vi "getlastmondata.vi"(0 "duplicate VISA resource name":refnum<visa-resource-name>, 1 "error out 2":errorcluster) -> (2 "duplicate VISA resource name 2":refnum<visa-resource-name>, 3 "output cluster":T1, 4 "N":u16, 5 "error out":errorcluster)   [LabVIEW 2010]
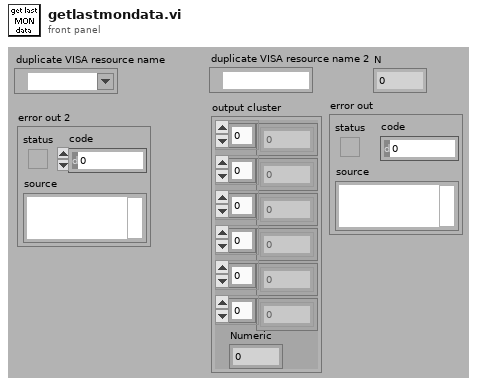
[diagram p1: front panel]
types:
  T1 = cluster{u16[], u16[], u16[], u16[], u16[], u16[], "Numeric":dbl}
  T2 = cluster{u16[], u16[], u16[], u16[], u16[], u16[], u16}
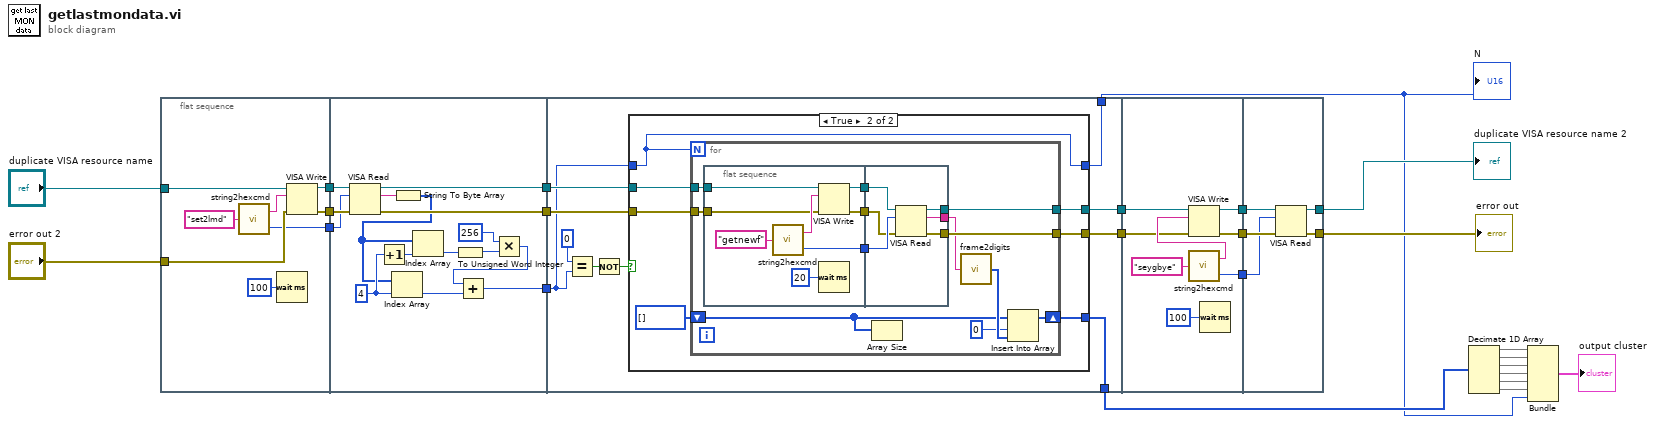
[diagram p0: block diagram]
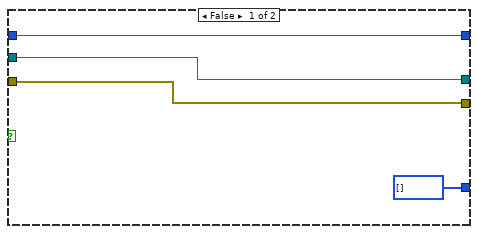
[diagram p2: hidden frame]
diagram:
  n1 = flat-sequence {
    tunnel: "duplicate VISA resource name" -> [w31]
    tunnel: [w29] -> w7
    tunnel: "error out 2" -> [w27]
    tunnel: [w26] -> w5
    tunnel: [w25] -> w3
    tunnel: w7 -> [w44]
    tunnel: [w47] -> w6
    tunnel: w5 -> [w45]
    tunnel: [w46] -> w4
    tunnel: w3 -> [w43]
    tunnel: [w33] -> w2
    tunnel: w6 -> [w57]
    tunnel: w4 -> [w56]
    tunnel: [w55] -> w24
    tunnel: [w54] -> w23
    tunnel: [w53] -> w8
    tunnel: w2 -> [w51]
    tunnel: [w48] -> w1
    tunnel: [w101] -> w22
    tunnel: [w100] -> w21
    tunnel: [w97] -> w20
    tunnel: w24 -> [w95]
    tunnel: w23 -> [w96]
    tunnel: w22 -> [w104]
    tunnel: w21 -> [w107]
    tunnel: w20 -> [w106]
    tunnel: [w105] -> w9
    tunnel: [w103] -> w12
    frame #0 {
      n2 = call "string2hexcmd.vi"("String comand"="set2lmd") -> ("hex comand"=w30:string, "byte count"=w25:u32)
      n3 = Wait (ms)(milliseconds to wait=u32 100) -> ()  [unwired: 1 out]
      n4 = VISA Write(VISA resource name=w31, write buffer=w30, error in (no error)=w27) -> (VISA resource name out=w29:refnum<visa-resource-name>, error out=w26:errorcluster)  [unwired: 1 out]
    }
    frame #1 {
      w40 = 4 ("index")
      n5 = VISA Read(VISA resource name=w44, byte count=w43, error in (no error)=w45) -> (VISA resource name out=w47:refnum<visa-resource-name>, read buffer=w42:string, error out=w46:errorcluster)  [unwired: 1 out]
      n6 = Increment(x=w40) -> (x+1=w41:i32)
      n7 = String To Byte Array(string=w42) -> (unsigned byte array=w38:u8[])
      n8 = Index Array(array=w38, index=w40) -> (element=w34:u8)
      n9 = Index Array(array=w38, index=w41) -> (element=w39:u8)
      n10 = To Unsigned Word Integer(number=w39) -> (unsigned 16bit integer=w36:u16)
      n11 = Multiply(x=u16 256, y=w36) -> (x*y=w35:u16)
      n12 = Add(x=w35, y=w34) -> (x+y=w33:u16)
    }
    frame #2 {
      n13 = Equal?(x=0, y=w51) -> (x = y?=w50:bool)
      n14 = Not(x=w50) -> (.not. x?=w49:bool)
      n15 = case shown="True" w49 {
        tunnel: w57 -> [w61 w68]
        tunnel: w56 -> [w60 w67]
        tunnel: [w60 w66] -> w55
        tunnel: [w61 w65] -> w54
        tunnel: [u16[] [] ("Digits") w62] -> w53
        tunnel: w51 -> [w58 w64]
        tunnel: [w58 w64] -> w48
        frame False {
        }
        frame True {
          n16 = for {
            N: w64 -> [_]
            tunnel: [w77] -> w65
            tunnel: [w76] -> w66
            tunnel: w68 -> [w75]
            tunnel: w67 -> [w74]
            shift-right: [w72] -> w62
            shift-left: u16[] [] -> [w70]
            n17 = flat-sequence {
              tunnel: [w85] -> w80
              tunnel: [w84] -> w79
              tunnel: [w83] -> w78
              tunnel: w75 -> [w82]
              tunnel: w74 -> [w81]
              tunnel: w80 -> [w94]
              tunnel: w79 -> [w93]
              tunnel: w78 -> [w92]
              tunnel: [w91] -> w76
              tunnel: [w90] -> w77
              tunnel: [w89] -> w73
              frame #0 {
                n18 = call "string2hexcmd.vi"("String comand"="getnewf") -> ("hex comand"=w87:string, "byte count"=w85:u32)
                n19 = VISA Write(VISA resource name=w82, write buffer=w87, error in (no error)=w81) -> (VISA resource name out=w83:refnum<visa-resource-name>, error out=w84:errorcluster)  [unwired: 1 out]
                n20 = Wait (ms)(milliseconds to wait=u32 20) -> ()  [unwired: 1 out]
              }
              frame #1 {
                n21 = VISA Read(VISA resource name=w92, byte count=w94, error in (no error)=w93) -> (VISA resource name out=w90:refnum<visa-resource-name>, read buffer=w89:string, error out=w91:errorcluster)  [unwired: 1 out]
              }
            }
            n22 = Array Size(array=w70) -> ()  [unwired: 1 out]
            n23 = call "frame2digits.vi"("data from COM Port"=w73) -> ("Digits"=w71:u16[])
            n24 = Insert Into Array(array=w70, index=0, new element=w71) -> (w72:u16[])
          }
        }
      }
    }
    frame #3 {
      n25 = call "string2hexcmd.vi"("String comand"="seygbye") -> ("hex comand"=w98:string, "byte count"=w101:u32)
      n26 = VISA Write(VISA resource name=w96, write buffer=w98, error in (no error)=w95) -> (VISA resource name out=w100:refnum<visa-resource-name>, error out=w97:errorcluster)  [unwired: 1 out]
      n27 = Wait (ms)(milliseconds to wait=u32 100) -> ()  [unwired: 1 out]
    }
    frame #4 {
      n28 = VISA Read(VISA resource name=w107, byte count=w104, error in (no error)=w106) -> (VISA resource name out=w103:refnum<visa-resource-name>, error out=w105:errorcluster)  [unwired: 2 out]
    }
  }
  n29 = Decimate 1D Array(w8) -> (w13:u16[], w14:u16[], w15:u16[], w16:u16[], w17:u16[], w18:u16[])
  n30 = Bundle(w13, w14, w15, w16, w17, w18, w1) -> (→"output cluster":T2)  [unwired: 1 in]
  "error out" <- w9
  "duplicate VISA resource name 2" <- w12
  "N" <- w1
